vi "ADCP_Processed_To_Raw_Packet.vi"(8 "error in (no error)":errorcluster, 10 "Processed Packet":u8[](array[numeric])=[0, 0, 0, 0, 0, 0, 0, 0, 0], 11 "ADCP in":refnum<class "ADCP.lvclass">) -> (0 "error out":errorcluster, 2 "Raw Packet":u8[](array[numeric]), 3 "ADCP out":refnum<class "ADCP.lvclass">)   [LabVIEW 2017, in "ADCP.lvclass"]
uses:
  ADCP.lvclass
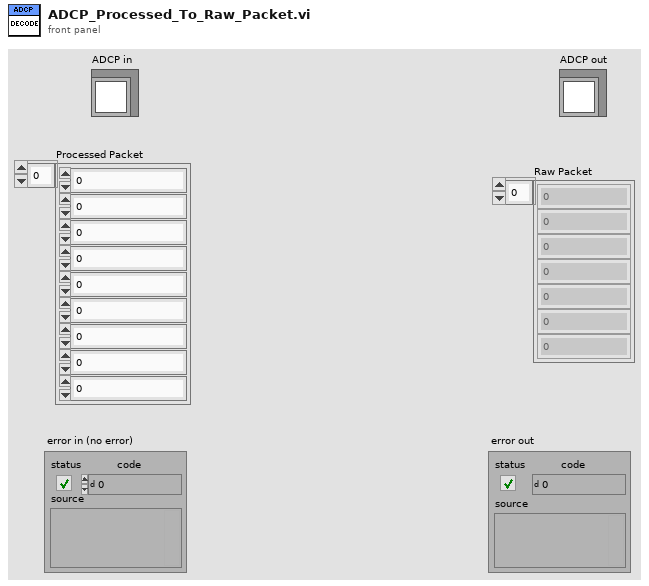
[diagram p1: front panel]
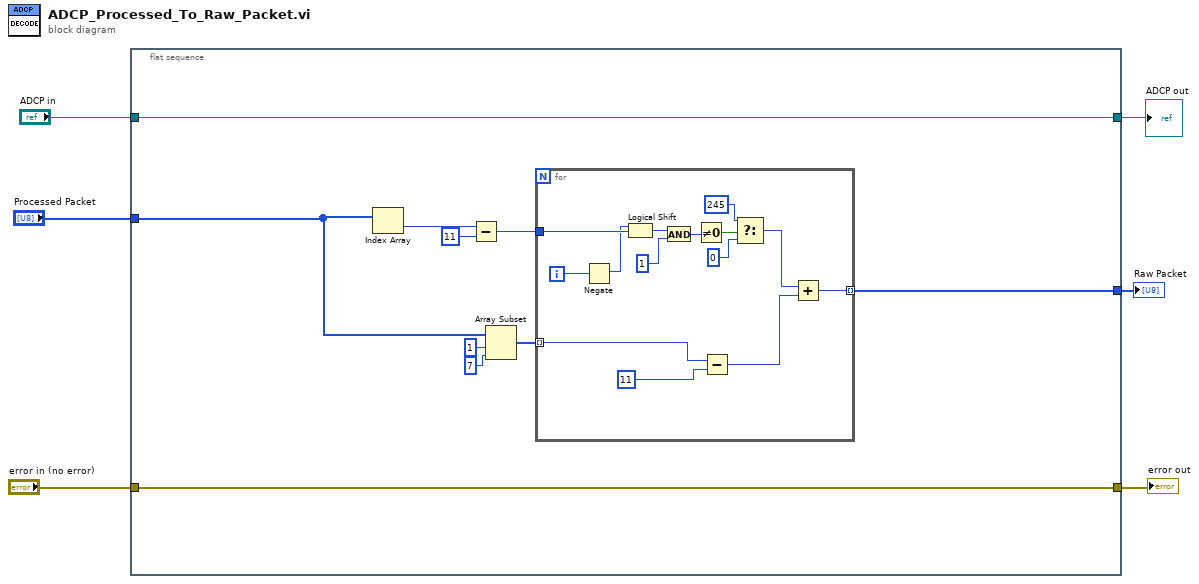
[diagram p0: block diagram]
diagram:
  n1 = flat-sequence {
    tunnel: "error in (no error)" -> [w16]
    tunnel: [w16] -> w5
    tunnel: "Processed Packet" -> [w9]
    tunnel: [w8] -> w3
    tunnel: "ADCP in" -> [w7]
    tunnel: [w7] -> w1
    frame #0 {
      n2 = Index Array(array=w9) -> (element=w15:u8)  [unwired: 1 in]
      n3 = Subtract(x=w15, y=u8 11) -> (x-y=w10:u8)
      n4 = Array Subset(array=w9, index=1, length=7) -> (w12:u8[])
      n5 = for {
        tunnel: w12 -> [w30] mode=indexing
        tunnel: [w24] -> w8 mode=indexing
        tunnel: w10 -> [w23]
        i -> [w22]
        n6 = Negate(x=w22) -> (-x=w21:i32)
        n7 = Logical Shift(y=w21, x=w23) -> (x << y=w20:u8)
        n8 = And(x=w20, y=u8 1) -> (x .and. y?=w18:u8)
        n9 = Not Equal To 0?(x=w18) -> (x != 0?=w17:bool)
        n10 = Subtract(x=w30, y=u8 11) -> (x-y=w25:u8)
        n11 = Select(t=u8 245 ("y"), s=w17, f=u8 0) -> (s? t:f=w26:u8)
        n12 = Add(x=w26, y=w25) -> (x+y=w24:u8)
      }
    }
  }
  "error out" <- w5
  "Raw Packet" <- w3
  "ADCP out" <- w1
